vi "Test Set Named Range.vi"(11 "Test Case In":refnum<class "Test Open Xml.lvclass">) -> (0 "error out":errorcluster, 3 "Test Case Out":refnum<class "Test Open Xml.lvclass">)   [LabVIEW 2025, in "Test Open Xml.lvclass"]
uses:
  Test Open Xml.lvclass
  <vilib>/Astemes/LUnit/Test Case.lvclass/Test Case.ctl
  81418309-5f46-498f-961d-c858d42f9635.vi
  <vilib>/Astemes/LUnit/Append Pass Result.vi
  <vilib>/Astemes/LUnit/Append Fail Result.vi
  81418309-5f46-498f-961d-c858d42f9635.vi/9c5d11cd-9439-4240-a1ee-d9baace9c924.vi
  <vilib>/Astemes/LUnit/Run In UI.vi
  <vilib>/Utility/error.llb/Clear Errors.vi
  Source/Open Xml.lvlib
panel:
  out "Sheet Name":string
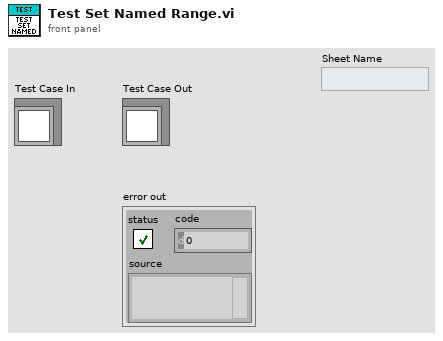
[diagram p1: front panel]
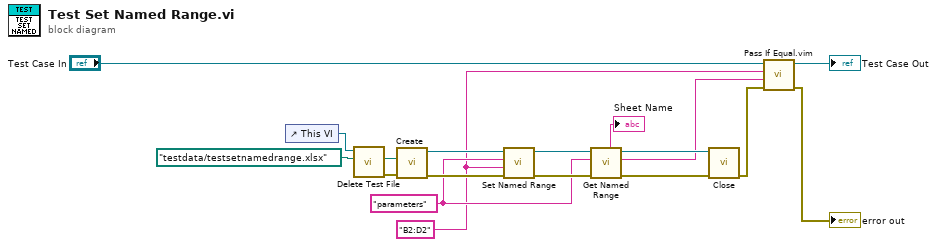
[diagram p0: block diagram]
diagram:
  w9 = "parameters" ("Range Identifier")
  w7 = "B2:D2" ("Range Identifier")
  n1 = control-ref of="This VI"() -> (w3:refnum<vi>)
  n2 = call "Delete Test File.vi"("name or relative path"=path "testdata/testsetnamedrange.xlsx", "VI in"=w3) -> ("error out"=w4:errorcluster, "deleted path"=w1:path)  [unwired: 8 in]
  n3 = call "Create.vi"("error in"=w4, "Path"=w1) -> ("error out"=w15:errorcluster, "SpreadsheetDoc"=w13:refnum<k24>)  [unwired: 8 in]
  n4 = call "Set Named Range.vi"("error in"=w15, "Cell Range"=w7, "Range Identifier"=w9, "SpreadsheetDoc in"=w13) -> ("error out"=w14:errorcluster, "SpreadsheetDoc out"=w11:refnum<k24>)  [unwired: 6 in]
  n5 = call "Get Named Range.vi"("error in"=w14, "Range Identifier"=w9, "SpreadsheetDoc in"=w11) -> ("error out"=w12:errorcluster, "Range"=w6:string, "SpreadsheetDoc out"=w10:refnum<k24>, "Sheet Name"=→"Sheet Name":string)  [unwired: 5 in]
  n6 = call "Close.vi"("error in"=w12, "SpreadsheetDoc"=w10) -> ("error out"=w8:errorcluster)  [unwired: 9 in]
  n7 = call "Pass If Equal.vim"("error in (no error)"=w8, "Actual"=w6, "Expected"=w7, "LUnit Test Case In"="Test Case In") -> ("error out"=→"error out":errorcluster, "LUnit Test Case Out"=→"Test Case Out":refnum<class "Test Open Xml.lvclass">)  [unwired: 6 in]
